vi "DeviceWrite.vi"(4 "error in (no error)":errorcluster, 5 "Command":string, 7 "CmdLib In":refnum<k24>) -> (0 "error out":errorcluster, 3 "CmdLib Out":refnum<k24>)   [LabVIEW 2013]
uses:
  C:/Code/Apps/Utilities/AG-UC2-UC8/AG-UC2-UC8/Install/Samples/LabVIEW/LabVIEW 2013/CmdLibAgilis.dll
  CmdLibAgilis.dll
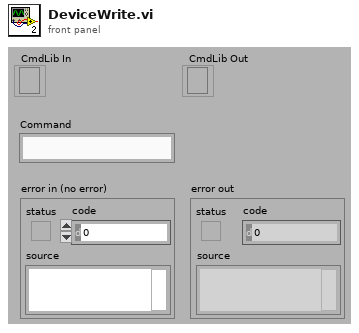
[diagram p1: front panel]
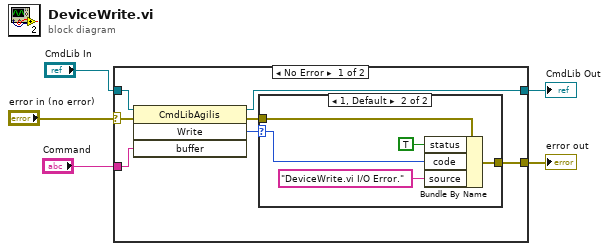
[diagram p0: block diagram]
diagram:
  n1 = case shown="No Error" "error in (no error)" {
    selector: "error in (no error)" -> [w7 w20]
    tunnel: [w9 w20] -> w4
    tunnel: "Command" -> [w6 _]
    tunnel: "CmdLib In" -> [w12 w19]
    tunnel: [w11 w19] -> w1
    frame No Error {
      n2 = invoke class="CmdLibAgilis" method="Write"(reference=w12, error in=w7, "buffer"=w6) -> (reference out=w11:refnum<k24>, error out=w8:errorcluster, "Write"=w10:i32)  [unwired: 1 in, 1 out]
      n3 = case shown="1, Default" w10 {
        selector: w10 -> [_ w14]
        tunnel: w8 -> [w13 w16]
        tunnel: [w13 w15] -> w9
        frame 0 {
        }
        frame 1, Default {
          n4 = Bundle By Name(cluster=w16, "status"=TRUE, "code"=w14, "source"="DeviceWrite.vi I/O Error.") -> (w15:errorcluster)
        }
      }
    }
    frame Error {
    }
  }
  "error out" <- w4
  "CmdLib Out" <- w1
